vi "Log.vi"(0 "object in":refnum<class "Excel.lvclass">, 2 "Requirements":T2, 5 "Error In":errorcluster) -> (14 "object out":refnum<class "Excel.lvclass">, 16 "Message":T1, 19 "Error Out":errorcluster)   [LabVIEW 2024, in "Excel.lvclass"]
doc: "Open or grap already existing Excel file and runs Logger classes Execute method"
uses:
  Excel.lvclass
  C:/Users/burakkorkmaz/Desktop/Leveling/labview-desing-patterns/Bridge Pattern/Abstractions/DataType/DataType.lvclass
  Support/Type Def/Requirements.ctl
  Support/Type Def/Message.ctl
  IDataMethod_interface/IDataMethod.lvclass
  Excel.lvclass/Excel.ctl
panel:
  # "Connector Pane"
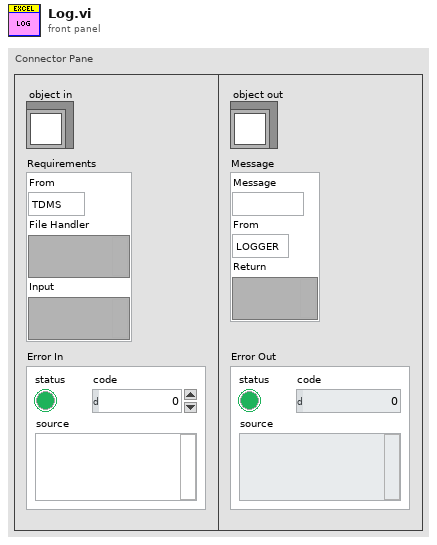
[diagram p1: front panel]
types:
  T1 = typedef "Message.ctl" = cluster{"Message":string, "From":enum16{"LOGGER", "VIEWER"}, "Return":variant}
  T2 = typedef "Requirements.ctl" = cluster{"From":enum16{"TDMS", "EXCEL"}, "File Handler":variant, "Input":variant}
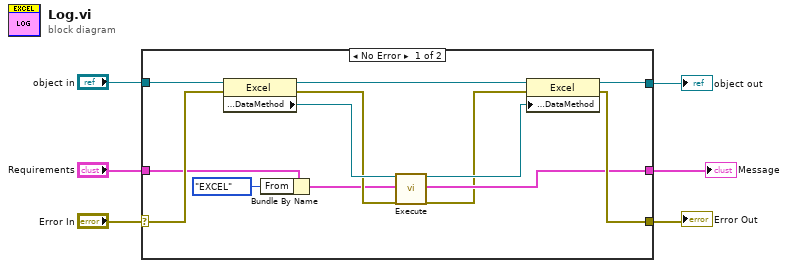
[diagram p0: block diagram]
diagram:
  n1 = case shown="No Error" "Error In" {
    selector: "Error In" -> [w16 w21]
    tunnel: [w15 w21] -> w5
    tunnel: [w17 w20] -> w3
    tunnel: "object in" -> [w19 w20]
    tunnel: "Requirements" -> [w14 _]
    tunnel: [w9 _] -> w1
    frame No Error {
      n2 = property class="Excel"(reference=w19, error in=w16) -> (reference out=w18:refnum<class "Excel.lvclass">, error out=w11:errorcluster, "properties:DataMethod"=w12:refnum<class "IDataMethod.lvclass">)
      n3 = Bundle By Name(cluster=w14, "From"=enum16{"TDMS", "EXCEL"}."EXCEL") -> (w10:T2)
      n4 = call-dynamic "Execute.vi"("object in"=w12, "Requirements"=w10, "Error In"=w11) -> ("object out"=w8:refnum<class "IDataMethod.lvclass">, "Message"=w9:T1, "Error Out"=w7:errorcluster)  [unwired: 14 in]
      n5 = property class="Excel"(reference=w18, error in=w7, "properties:DataMethod"=w8) -> (reference out=w17:refnum<class "Excel.lvclass">, error out=w15:errorcluster)
    }
    frame Error {
    }
  }
  "Error Out" <- w5
  "object out" <- w3
  "Message" <- w1
